vi "Read Wheel State.vi"(8 "error in (no error)":errorcluster, 10 "wheel state in":T1, 11 "steering wheel in":refnum<class "NI_Robotics_Steering Wheel.lvclass">) -> (0 "error out":errorcluster, 2 "wheel state out":T1, 3 "steering wheel out":refnum<class "NI_Robotics_Steering Wheel.lvclass">)   [LabVIEW 2017, in "NI_Robotics_Steering Wheel.lvclass"]
uses:
  <vilib>/robotics/Steering/Steering Wheel/NI_Robotics_Steering Wheel.lvclass
  <vilib>/robotics/Steering/Wheel/Wheel State.ctl
  <vilib>/robotics/Steering/Steering Wheel/NI_Robotics_Steering Wheel.lvclass/NI_Robotics_Steering Wheel.ctl
  <vilib>/robotics/Actuation/Motor Communication/Get Motor Angle State.vi
  <vilib>/robotics/Actuation/Motor Communication/Check if Valid.vi
  <vilib>/robotics/Utilities/Generate Error.vi
  <vilib>/robotics/Steering/Wheel/NI_Robotics_Wheel.lvclass
  <vilib>/robotics/Actuation/Motor Communication/NI_Robotics_Motor Communication.lvclass
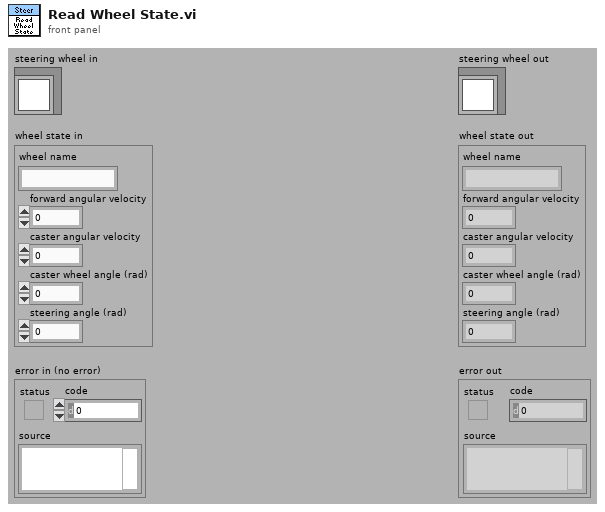
[diagram p1: front panel]
types:
  T1 = typedef "NI_Robotics_Wheel.lvclass/Wheel State.ctl" = cluster{"wheel name":string, "forward angular velocity":dbl, "caster angular velocity":dbl, "caster wheel angle (rad)":dbl, "steering angle (rad)":dbl}
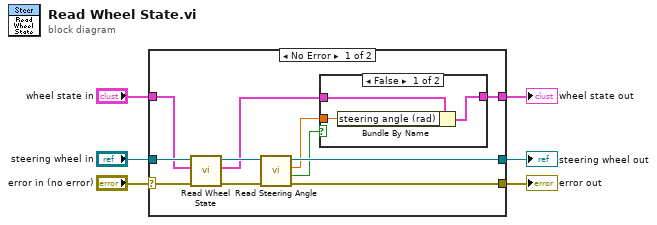
[diagram p0: block diagram]
diagram:
  n1 = case shown="No Error" "error in (no error)" {
    selector: "error in (no error)" -> [w16 w23]
    tunnel: [w12 w23] -> w6
    tunnel: [w10 w22] -> w5
    tunnel: [w14 w24] -> w4
    tunnel: "steering wheel in" -> [w17 w24]
    tunnel: "wheel state in" -> [w8 w22]
    frame No Error {
      n2 = call-parent "Read Wheel State.vi"("error in (no error)"=w16, "wheel state in"=w8, "wheel in"=w17) -> ("error out"=w13:errorcluster, "wheel state out"=w11:T1, "wheel out"=w15:refnum<class "NI_Robotics_Steering Wheel.lvclass">)  [unwired: 6 in]
      n3 = call <vilib>:"Read Steering Angle.vi"("error in (no error)"=w13, "steering wheel in"=w15) -> ("error out"=w12:errorcluster, "failed"=w7:bool, "steering angle (rad)"=w9:dbl, "steering wheel out"=w14:refnum<class "NI_Robotics_Steering Wheel.lvclass">)  [unwired: 6 in]
      n4 = case shown="False" w7 {
        tunnel: w11 -> [w20 w21]
        tunnel: [w19 w21] -> w10
        tunnel: w9 -> [w18 _]
        frame False {
          n5 = Bundle By Name(cluster=w20, "steering angle (rad)"=w18) -> (w19:T1)
        }
        frame True {
        }
      }
    }
    frame Error {
    }
  }
  "error out" <- w6
  "steering wheel out" <- w4
  "wheel state out" <- w5
